vi "recipe_wrapper.vi"(7 "references":T1, 8 "error in (no error)":errorcluster) -> (0 "error out":errorcluster)   [LabVIEW 2015, in "repub-dvr_nre.lvlib"]
uses:
  repub-dvr_nre.lvlib
  public/_controls/references.ctl
  _controls/input.ctl
  _controls/input_command.ctl
  _controls/output.ctl
  _controls/data.ctl
  public/_controls/configuration.ctl
  lv-recipe-machine/private/_controls/recipe_data.ctl
  lv-recipe-machine/public/_controls/mode.ctl
  lv-recipe-machine/public/_controls/manual_state.ctl
  lv-recipe-machine/public/_controls/automatic_state.ctl
  <userlib>/antonio-alexander/lv-waitgroup/public/_controls/api_waitgroup.ctl
  lv-recipe-machine/public/_controls/transition.ctl
  public/_controls/change.ctl
  lv-recipe-machine/lv-recipe-machine.lvlib
  <userlib>/antonio-alexander/lv-waitgroup/lv-waitgroup.lvlib
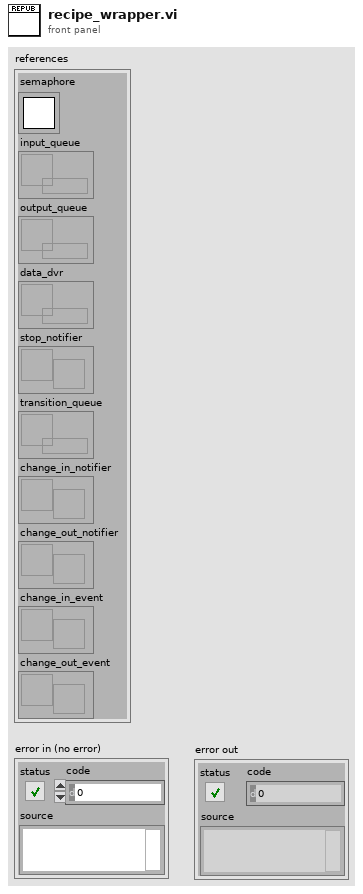
[diagram p1: front panel]
types:
  T1 = typedef "repub-dvr_nre.lvlib/references.ctl" = cluster{"semaphore":T2, "input_queue":refnum<queue>, "output_queue":refnum<queue>, "data_dvr":refnum<data-value>, "stop_notifier":refnum<notifier>, "transition_queue":refnum<queue>, "change_in_notifier":refnum<notifier>, "change_out_notifier":refnum<notifier>, "change_in_event":refnum<user-event>, "change_out_event":refnum<user-event>}
  T2 = typedef "Semaphore RefNum" = refnum<k1>
  T3 = typedef "repub-dvr_nre.lvlib/data.ctl" = cluster{"configuration":T4, "working":cluster{"recipe_data":T5, "api_waitgroup":T9}}
  T4 = typedef "repub-dvr_nre.lvlib/configuration.ctl" = cluster{dbl}
  T5 = typedef "lv-recipe-machine.lvlib/recipe_data.ctl" = cluster{"mode":T6, "manual_state":T7, "automatic_state":T8, "step":string, "automatic_recipe":variant, "manual_actions":variant}
  T6 = typedef "lv-recipe-machine.lvlib/mode.ctl" = enum16{"<mode>", "manual", "automatic", "<null>"}
  T7 = typedef "lv-recipe-machine.lvlib/manual_state.ctl" = enum16{"<manual_state>", "failed", "action", "running", "idle", "<null>"}
  T8 = typedef "lv-recipe-machine.lvlib/automatic_state.ctl" = enum16{"<automatic_state>", "failed", "idle", "running", "paused", "transition", "stopped", "<null>"}
  T9 = typedef "lv-waitgroup.lvlib/api_waitgroup.ctl" = cluster{"waitgroups":refnum<data-value>, "waitgroup":string}
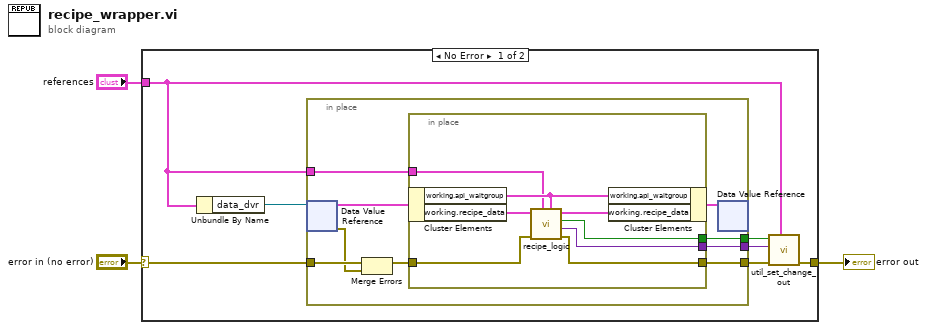
[diagram p0: block diagram]
diagram:
  n1 = case shown="No Error" "error in (no error)" {
    selector: "error in (no error)" -> [w10 w28]
    tunnel: [w8 w28] -> w2
    tunnel: "references" -> [w4 _]
    frame No Error {
      n2 = Unbundle By Name(w4) -> ("data_dvr"=w9:refnum<data-value>)
      n3 = in-place {
        in-place-border: w10 -> [w19]
        in-place-border: [w14] -> w7
        in-place-border: [w13] -> w6
        in-place-border: [w12] -> w5
        in-place-border: w4 -> [w11]
        n4 = in-place-dvr #1(w9) -> (w17:T3, w16:errorcluster)
        n5 = Merge Errors(w19, w16) -> (w18:errorcluster)
        n6 = in-place {
          in-place-border: w18 -> [w27]
          in-place-border: [w26] -> w14
          in-place-border: [w23] -> w13
          in-place-border: w11 -> [w21]
          in-place-border: [w20] -> w12
          n7 = in-place-cluster #2(w17) -> ("working.api_waitgroup"=w22:T9, "working.recipe_data"=w25:T5)
          n8 = call "recipe_logic.vi"("waitgroup"=w22, "references"=w21, "error in (no error)"=w27, "data_in"=w25) -> ("error out"=w26:errorcluster, "data"=w20:variant, "change"=w23:bool, "data_out"=w24:T5)  [unwired: 4 in]
          n9 = in-place-cluster #2("working.api_waitgroup"=w22, "working.recipe_data"=w24) -> (w15:T3)
        }
        n10 = in-place-dvr #1(w15) -> ()  [unwired: 2 out]
      }
      n11 = call "util_set_change_out.vi"("references"=w4, "error in (no error)"=w7, "data"=w5, "change"=w6) -> ("error out"=w8:errorcluster)  [unwired: 7 in]
    }
    frame Error {
    }
  }
  "error out" <- w2
